vi "VI Graph.vi"() -> ()   [LabVIEW 2020, in "Grafik.lvlib"]
uses:
  Grafik.lvlib
  Visualisierungs Elemente/Zahlen-Ausgabefeld.ctl
  Visualisierungs Elemente/Auswahlfeld.ctl
  Visualisierungs Elemente/Button.ctl
  Aktionen Konfig Diagramme.ctl
  FT-IR/FGV FT-IR Gasliste Aktionen.ctl
  Gaszuordnung AO/FGV Gaszuordnung Gas-Auswahl Aktion.ctl
  Messdaten/Aktionen FGV Messdaten.ctl
  FT-IR/FGV FT-IR Parameter.vi
  FT-IR/FT-IR.lvlib
  Messdaten/Messdaten.lvlib
  Allgemein/allgemeine Sub-VIs.lvlib
  Gaszuordnung AO/Gaszuordnung AO.lvlib
panel:
  in  "Zoom deaktivieren":T1 caption="Graphen löschen"
  out "Mwert 6":sgl format="%.3f"
  out "PMwert 6":sgl format="%.3f"
  out "Mwert 5":sgl format="%.3f"
  out "PMwert 5":sgl format="%.3f"
  out "Mwert 4":sgl format="%.3f"
  out "PMwert 4":sgl format="%.3f"
  out "Mwert 3":sgl format="%.3f"
  out "PMwert 3":sgl format="%.3f"
  out "Mwert 2":sgl format="%.3f"
  out "PMwert 2":sgl format="%.3f"
  out "Mwert":sgl format="%.3f"
  out "PMwert":sgl format="%.3f"
  in  "Graphen löschen":T1
  in  "Konfig":T1
  out "Wert 6":T2 caption="Konzentration" format="%#.3f"
  out "Wert 5":T2 caption="Konzentration" format="%#.3f"
  in  "Gas 6":T3=1 items=["NO (3000) LP 191C", "NO2 (150) LP 191C (1of2)", "NO2 (2000) LP 191C (2of2)", "N2O (300) LP 191C (1of2)", "NH3 (300) LP 191C (1of2)", "NH3 (900,3000) LP 191C (2of2)", "HNCO (400) 191C", "H2O% (30) LP 191C", "Formaldehyde (70,500) LP 191C", "CO2 low% (4) LP 191C (2of2)", "CO2% (20) LP 191C (1of2)", "CO (700) LP 191C (1of3)", "CO% (1) LP 191C (2of3)", "Propylene (1000) LP 191C", "Aromatic HC C7 (500) LP 191C", "Ethylene (1000) LP 191C", "CH4 (250) LP 191C (1of2)", "CH4 (5000) LP 191C (2of2)", "Ethane (1000) LP 191C", "Acetylene (1000) LP 191C", "HNO2 (20) 191C", "MeOH (1000) 191C", "CO% (10) LP 191C (3of3)", "Formic Acid (100) 191C", "SO2 (500) LP 191C", "Acetaldehyde (1000) LP 191C", "COS (100) LP 191C", "1,3 butadiene (100) LP 191C", "Oil as Octane (200) LP 191C", "N2O (1000) LP 191C (2of2)", "Propane (200) LP 191C", "NO2 autorange (2000)", "CO autorange (100000)", "CH4 autorange (5000)", "NH3 autorange (3000)", "NOx autorange (3000)", "HCD (10000)", "NMHCD (10000)", "CO2% autorange (20)", "H2Oppm (300000)", "N2O autorange (1000)", "NMNEHCD (3000)", "Temp. Gascell", "Pressure Gascell", "sBeam@2500", "Temp. HL to FT-IR", "Temp. HL Extern SP1", "Outlet Temp FT-IR", "Temp. Cabinet", "Constant 0", "Constant 50", "Constant 100", "AK DUMMY"]
  in  "Gas 5":T3=1 items=["NO (3000) LP 191C", "NO2 (150) LP 191C (1of2)", "NO2 (2000) LP 191C (2of2)", "N2O (300) LP 191C (1of2)", "NH3 (300) LP 191C (1of2)", "NH3 (900,3000) LP 191C (2of2)", "HNCO (400) 191C", "H2O% (30) LP 191C", "Formaldehyde (70,500) LP 191C", "CO2 low% (4) LP 191C (2of2)", "CO2% (20) LP 191C (1of2)", "CO (700) LP 191C (1of3)", "CO% (1) LP 191C (2of3)", "Propylene (1000) LP 191C", "Aromatic HC C7 (500) LP 191C", "Ethylene (1000) LP 191C", "CH4 (250) LP 191C (1of2)", "CH4 (5000) LP 191C (2of2)", "Ethane (1000) LP 191C", "Acetylene (1000) LP 191C", "HNO2 (20) 191C", "MeOH (1000) 191C", "CO% (10) LP 191C (3of3)", "Formic Acid (100) 191C", "SO2 (500) LP 191C", "Acetaldehyde (1000) LP 191C", "COS (100) LP 191C", "1,3 butadiene (100) LP 191C", "Oil as Octane (200) LP 191C", "N2O (1000) LP 191C (2of2)", "Propane (200) LP 191C", "NO2 autorange (2000)", "CO autorange (100000)", "CH4 autorange (5000)", "NH3 autorange (3000)", "NOx autorange (3000)", "HCD (10000)", "NMHCD (10000)", "CO2% autorange (20)", "H2Oppm (300000)", "N2O autorange (1000)", "NMNEHCD (3000)", "Temp. Gascell", "Pressure Gascell", "sBeam@2500", "Temp. HL to FT-IR", "Temp. HL Extern SP1", "Outlet Temp FT-IR", "Temp. Cabinet", "Constant 0", "Constant 50", "Constant 100", "AK DUMMY"]
  in  "Gas 2":T3=1 items=["NO (3000) LP 191C", "NO2 (150) LP 191C (1of2)", "NO2 (2000) LP 191C (2of2)", "N2O (300) LP 191C (1of2)", "NH3 (300) LP 191C (1of2)", "NH3 (900,3000) LP 191C (2of2)", "HNCO (400) 191C", "H2O% (30) LP 191C", "Formaldehyde (70,500) LP 191C", "CO2 low% (4) LP 191C (2of2)", "CO2% (20) LP 191C (1of2)", "CO (700) LP 191C (1of3)", "CO% (1) LP 191C (2of3)", "Propylene (1000) LP 191C", "Aromatic HC C7 (500) LP 191C", "Ethylene (1000) LP 191C", "CH4 (250) LP 191C (1of2)", "CH4 (5000) LP 191C (2of2)", "Ethane (1000) LP 191C", "Acetylene (1000) LP 191C", "HNO2 (20) 191C", "MeOH (1000) 191C", "CO% (10) LP 191C (3of3)", "Formic Acid (100) 191C", "SO2 (500) LP 191C", "Acetaldehyde (1000) LP 191C", "COS (100) LP 191C", "1,3 butadiene (100) LP 191C", "Oil as Octane (200) LP 191C", "N2O (1000) LP 191C (2of2)", "Propane (200) LP 191C", "NO2 autorange (2000)", "CO autorange (100000)", "CH4 autorange (5000)", "NH3 autorange (3000)", "NOx autorange (3000)", "HCD (10000)", "NMHCD (10000)", "CO2% autorange (20)", "H2Oppm (300000)", "N2O autorange (1000)", "NMNEHCD (3000)", "Temp. Gascell", "Pressure Gascell", "sBeam@2500", "Temp. HL to FT-IR", "Temp. HL Extern SP1", "Outlet Temp FT-IR", "Temp. Cabinet", "Constant 0", "Constant 50", "Constant 100", "AK DUMMY"]
  out "Wert 2":T2 caption="Konzentration" format="%#.3f"
  in  "Gas 4":T3=1 items=["NO (3000) LP 191C", "NO2 (150) LP 191C (1of2)", "NO2 (2000) LP 191C (2of2)", "N2O (300) LP 191C (1of2)", "NH3 (300) LP 191C (1of2)", "NH3 (900,3000) LP 191C (2of2)", "HNCO (400) 191C", "H2O% (30) LP 191C", "Formaldehyde (70,500) LP 191C", "CO2 low% (4) LP 191C (2of2)", "CO2% (20) LP 191C (1of2)", "CO (700) LP 191C (1of3)", "CO% (1) LP 191C (2of3)", "Propylene (1000) LP 191C", "Aromatic HC C7 (500) LP 191C", "Ethylene (1000) LP 191C", "CH4 (250) LP 191C (1of2)", "CH4 (5000) LP 191C (2of2)", "Ethane (1000) LP 191C", "Acetylene (1000) LP 191C", "HNO2 (20) 191C", "MeOH (1000) 191C", "CO% (10) LP 191C (3of3)", "Formic Acid (100) 191C", "SO2 (500) LP 191C", "Acetaldehyde (1000) LP 191C", "COS (100) LP 191C", "1,3 butadiene (100) LP 191C", "Oil as Octane (200) LP 191C", "N2O (1000) LP 191C (2of2)", "Propane (200) LP 191C", "NO2 autorange (2000)", "CO autorange (100000)", "CH4 autorange (5000)", "NH3 autorange (3000)", "NOx autorange (3000)", "HCD (10000)", "NMHCD (10000)", "CO2% autorange (20)", "H2Oppm (300000)", "N2O autorange (1000)", "NMNEHCD (3000)", "Temp. Gascell", "Pressure Gascell", "sBeam@2500", "Temp. HL to FT-IR", "Temp. HL Extern SP1", "Outlet Temp FT-IR", "Temp. Cabinet", "Constant 0", "Constant 50", "Constant 100", "AK DUMMY"]
  in  "Gas 1":T3 items=["NO (3000) LP 191C", "NO2 (150) LP 191C (1of2)", "NO2 (2000) LP 191C (2of2)", "N2O (300) LP 191C (1of2)", "NH3 (300) LP 191C (1of2)", "NH3 (900,3000) LP 191C (2of2)", "HNCO (400) 191C", "H2O% (30) LP 191C", "Formaldehyde (70,500) LP 191C", "CO2 low% (4) LP 191C (2of2)", "CO2% (20) LP 191C (1of2)", "CO (700) LP 191C (1of3)", "CO% (1) LP 191C (2of3)", "Propylene (1000) LP 191C", "Aromatic HC C7 (500) LP 191C", "Ethylene (1000) LP 191C", "CH4 (250) LP 191C (1of2)", "CH4 (5000) LP 191C (2of2)", "Ethane (1000) LP 191C", "Acetylene (1000) LP 191C", "HNO2 (20) 191C", "MeOH (1000) 191C", "CO% (10) LP 191C (3of3)", "Formic Acid (100) 191C", "SO2 (500) LP 191C", "Acetaldehyde (1000) LP 191C", "COS (100) LP 191C", "1,3 butadiene (100) LP 191C", "Oil as Octane (200) LP 191C", "N2O (1000) LP 191C (2of2)", "Propane (200) LP 191C", "NO2 autorange (2000)", "CO autorange (100000)", "CH4 autorange (5000)", "NH3 autorange (3000)", "NOx autorange (3000)", "HCD (10000)", "NMHCD (10000)", "CO2% autorange (20)", "H2Oppm (300000)", "N2O autorange (1000)", "NMNEHCD (3000)", "Temp. Gascell", "Pressure Gascell", "sBeam@2500", "Temp. HL to FT-IR", "Temp. HL Extern SP1", "Outlet Temp FT-IR", "Temp. Cabinet", "Constant 0", "Constant 50", "Constant 100", "AK DUMMY"]
  out "Wert 1":T2 caption="Konzentration" format="%#.3f"
  out "Wert 4":T2 caption="Konzentration" format="%#.3f"
  out "Wert 3":T2 caption="Konzentration" format="%#.3f"
  in  "Gas 3":T3=1 items=["NO (3000) LP 191C", "NO2 (150) LP 191C (1of2)", "NO2 (2000) LP 191C (2of2)", "N2O (300) LP 191C (1of2)", "NH3 (300) LP 191C (1of2)", "NH3 (900,3000) LP 191C (2of2)", "HNCO (400) 191C", "H2O% (30) LP 191C", "Formaldehyde (70,500) LP 191C", "CO2 low% (4) LP 191C (2of2)", "CO2% (20) LP 191C (1of2)", "CO (700) LP 191C (1of3)", "CO% (1) LP 191C (2of3)", "Propylene (1000) LP 191C", "Aromatic HC C7 (500) LP 191C", "Ethylene (1000) LP 191C", "CH4 (250) LP 191C (1of2)", "CH4 (5000) LP 191C (2of2)", "Ethane (1000) LP 191C", "Acetylene (1000) LP 191C", "HNO2 (20) 191C", "MeOH (1000) 191C", "CO% (10) LP 191C (3of3)", "Formic Acid (100) 191C", "SO2 (500) LP 191C", "Acetaldehyde (1000) LP 191C", "COS (100) LP 191C", "1,3 butadiene (100) LP 191C", "Oil as Octane (200) LP 191C", "N2O (1000) LP 191C (2of2)", "Propane (200) LP 191C", "NO2 autorange (2000)", "CO autorange (100000)", "CH4 autorange (5000)", "NH3 autorange (3000)", "NOx autorange (3000)", "HCD (10000)", "NMHCD (10000)", "CO2% autorange (20)", "H2Oppm (300000)", "N2O autorange (1000)", "NMNEHCD (3000)", "Temp. Gascell", "Pressure Gascell", "sBeam@2500", "Temp. HL to FT-IR", "Temp. HL Extern SP1", "Outlet Temp FT-IR", "Temp. Cabinet", "Constant 0", "Constant 50", "Constant 100", "AK DUMMY"]
  out "Graph1":waveform(dbl)[](graph)
  out "Graph 3":waveform(dbl)[](graph)
  out "Graph 2":waveform(dbl)[](graph)
  out "Graph 4":waveform(dbl)[](graph)
  out "Graph 6":waveform(dbl)[](graph)
  out "Graph 5":waveform(dbl)[](graph)
  # "Grafik"
  # "Grafik 4"
  # "Grafik 1"
  # "Grafik 2"
  # "Grafik 5"
  # "Grafik 6"
  # "Grafik 3"
  # "±"
  # "x"
  # "±"
  # "x"
  # "±"
  # "x"
  # "±"
  # "x"
  # "±"
  # "x"
  # "±"
  # "x"
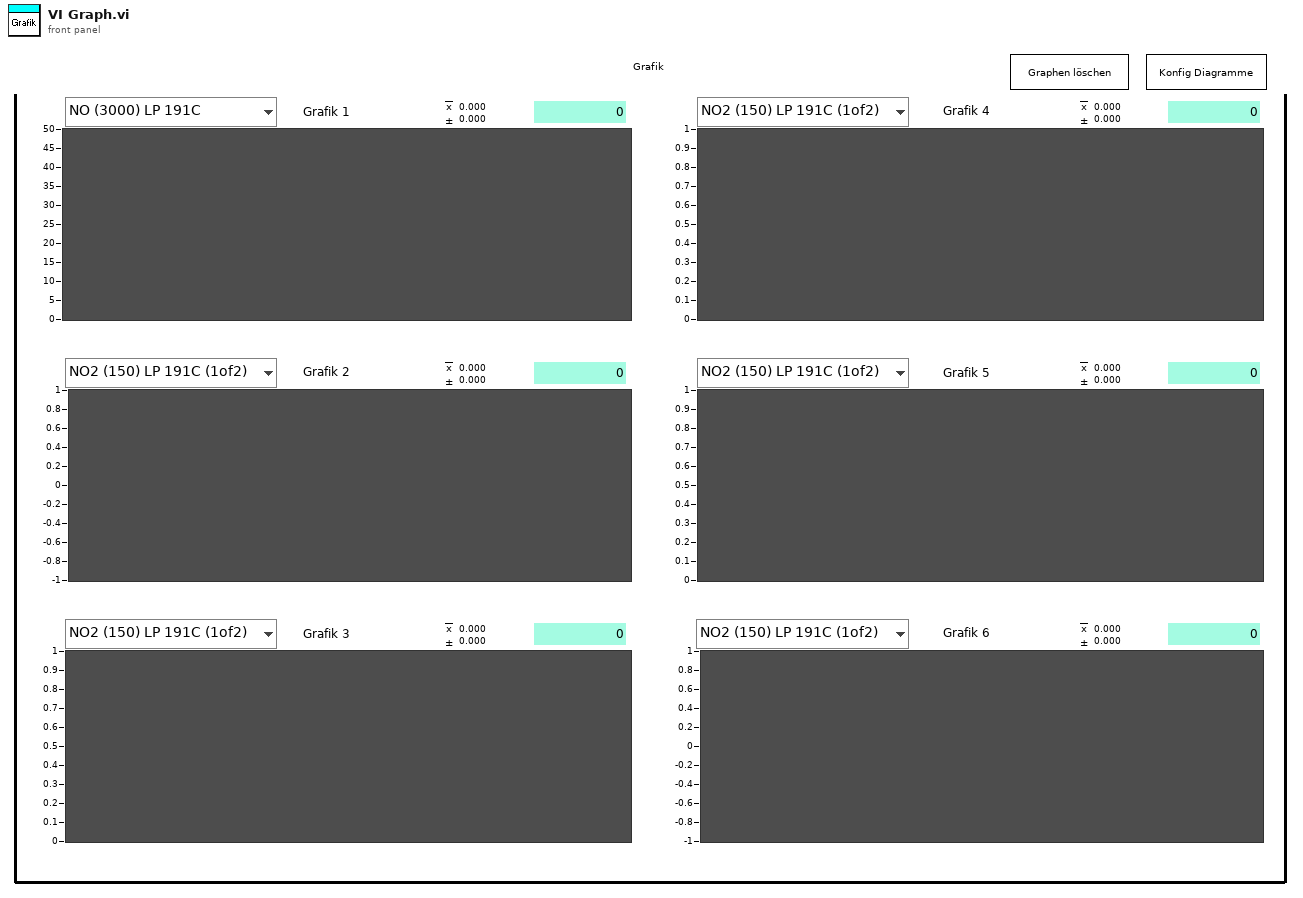
[diagram p1: front panel]
types:
  T1 = typedef "Button.ctl" = bool
  T2 = typedef "Zahlen-Ausgabefeld.ctl" = sgl
  T3 = typedef "Auswahlfeld.ctl" = u16
  T4 = typedef "Gaszuordnung AO.lvlib/FGV Gaszuordnung Gas-Auswahl Aktion.ctl" = enum16{"Lesen", "AO Auswahl", "Graph Auswahl", "aktiver Graph", "laden", "speichern"}
  T5 = typedef "FT-IR.lvlib/FGV FT-IR Gasliste Aktionen.ctl" = enum16{"lesen", "Gasliste FT-IR", "Gasliste ausgelesen", "laden", "speichern", "löschen"}
  T6 = typedef "Grafik.lvlib/Aktionen Konfig Diagramme.ctl" = enum16{"lesen", "laden", "speichern", "X Auto Scale", "Y Auto Scale", "Anzeigedauer", "Y MIN", "Y MAX", "Referenzen", "Werteanzahl", "Autoscale einzeln"}
  T7 = typedef "Zahlen-Eingabefeld.ctl" = sgl
  T8 = cluster{"Y Anzeige MIN 1":T7, "Y Anzeige MIN 2":T7, "Y Anzeige MIN 3":T7, "Y Anzeige MIN 4":T7, "Y Anzeige MIN 5":T7, "Y Anzeige MIN 6":T7}
  T9 = cluster{"Y Anzeige MAX 1":T7, "Y Anzeige MAX 2":T7, "Y Anzeige MAX 3":T7, "Y Anzeige MAX 4":T7, "Y Anzeige MAX 5":T7, "Y Anzeige MAX 6":T7}
  T10 = typedef "String - Ausgabefeld.ctl" = string
  T11 = typedef "Grafik.lvlib/Graphen Auswahl.ctl" = u16[]
  T12 = cluster{"Graphen[0]":u16, "Graphen[1]":u16, "Graphen[2]":u16, "Graphen[3]":u16, "Graphen[4]":u16, "Graphen[5]":u16}
  T13 = typedef "Messdaten.lvlib/Aktionen FGV Messdaten.ctl" = enum16{"lesen", "schreiben", "löschen", "Mittelwerte", "Komponente"}
  T14 = cluster{"[0]":waveform(dbl), "[1]":waveform(dbl), "[2]":waveform(dbl)}
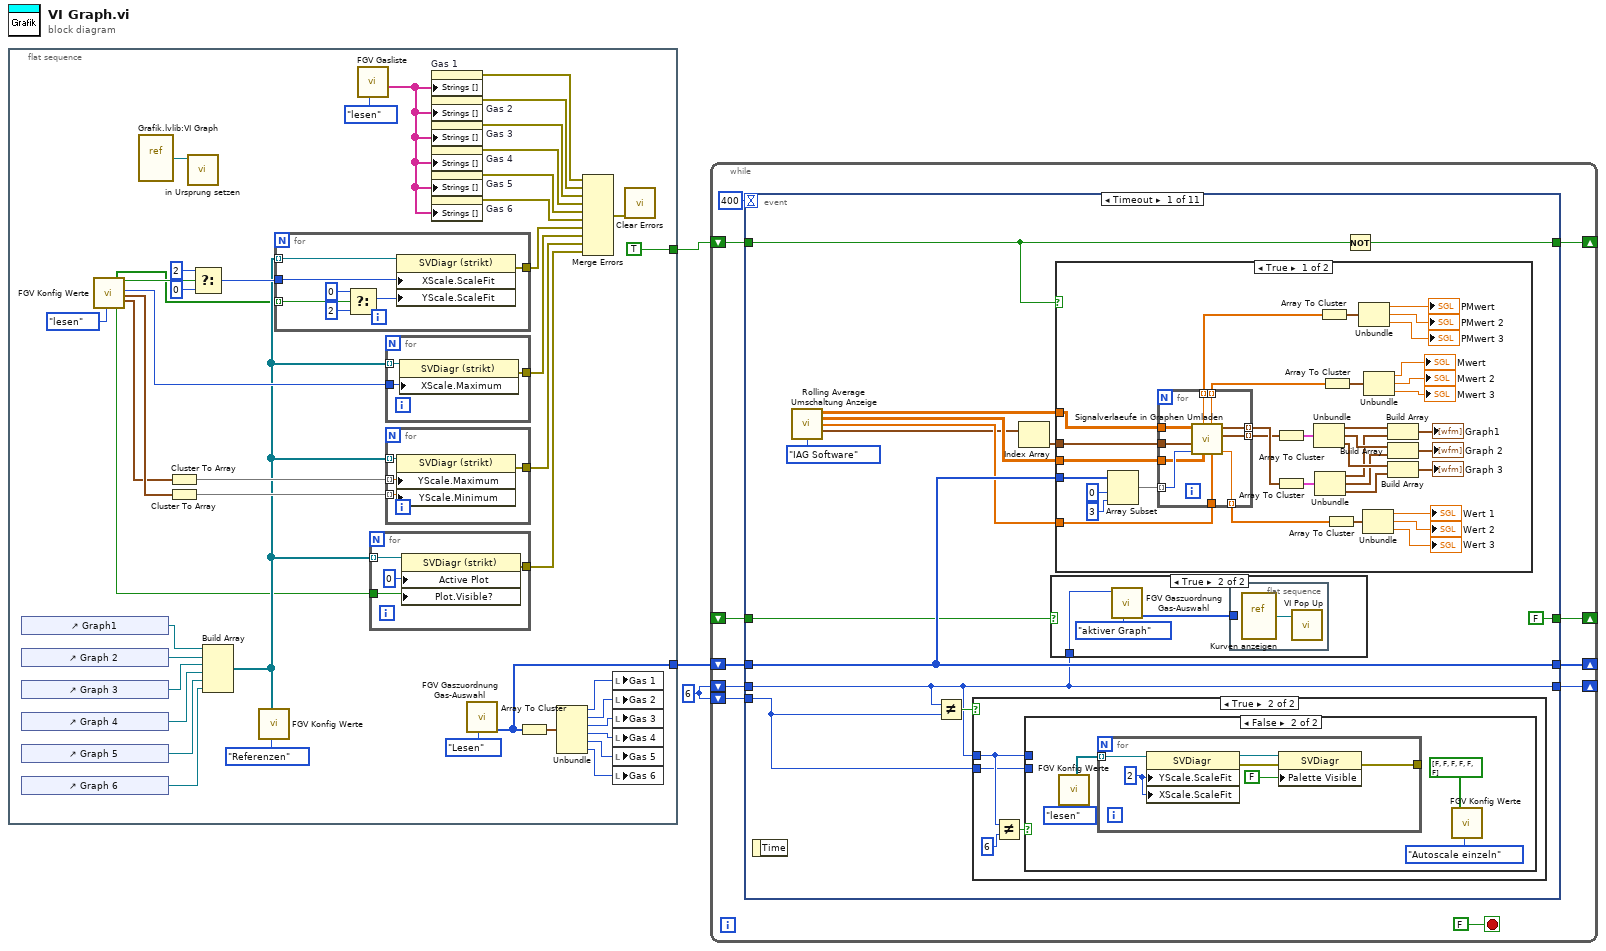
[diagram p0: block diagram]
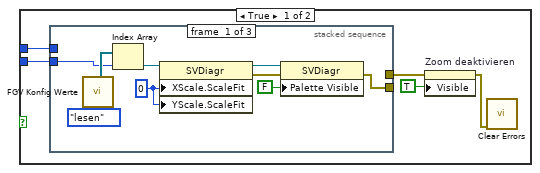
[diagram p4: hidden frame]
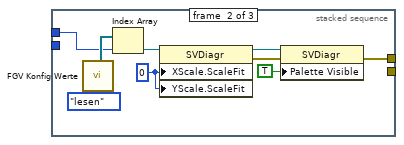
[diagram p5: hidden frame]
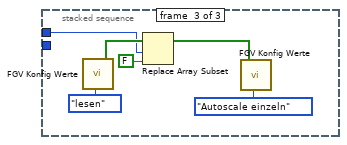
[diagram p6: hidden frame]
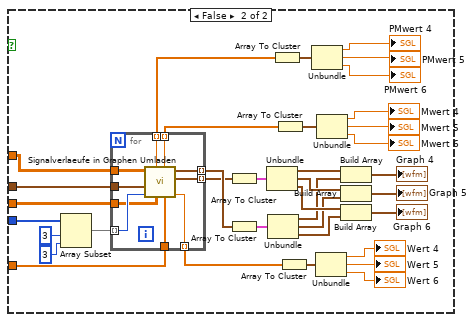
[diagram p7: hidden frame]
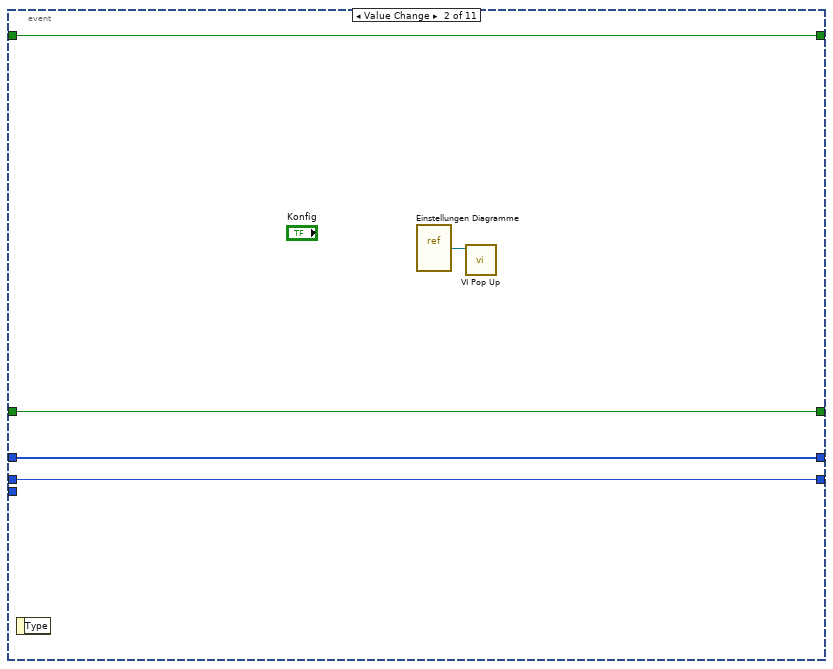
[diagram p8: hidden frame]
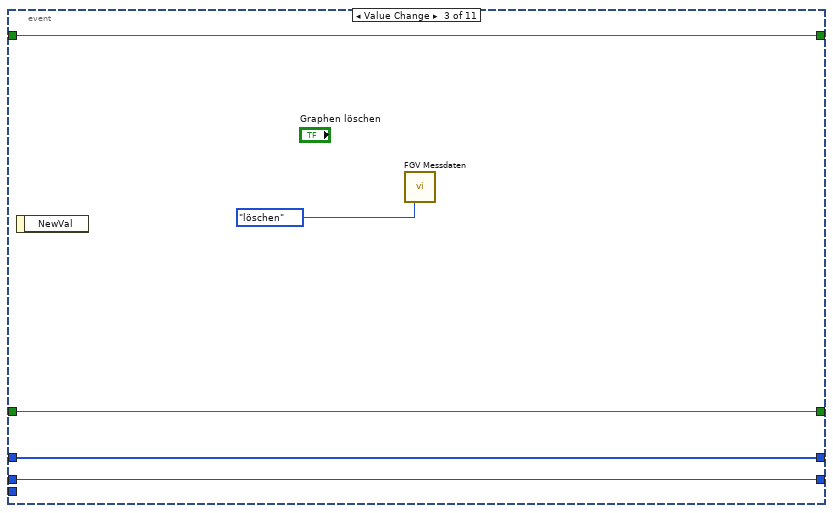
[diagram p9: hidden frame]
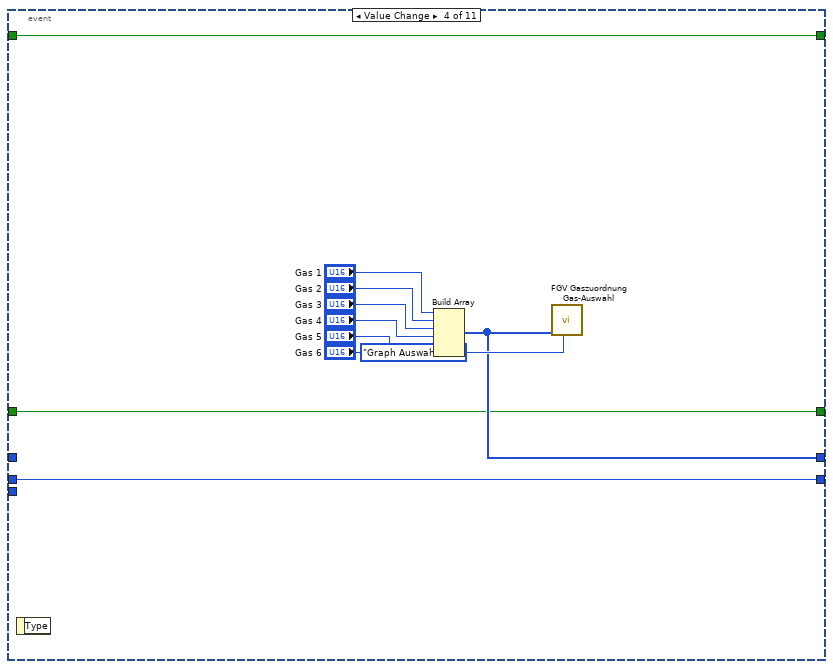
[diagram p10: hidden frame]
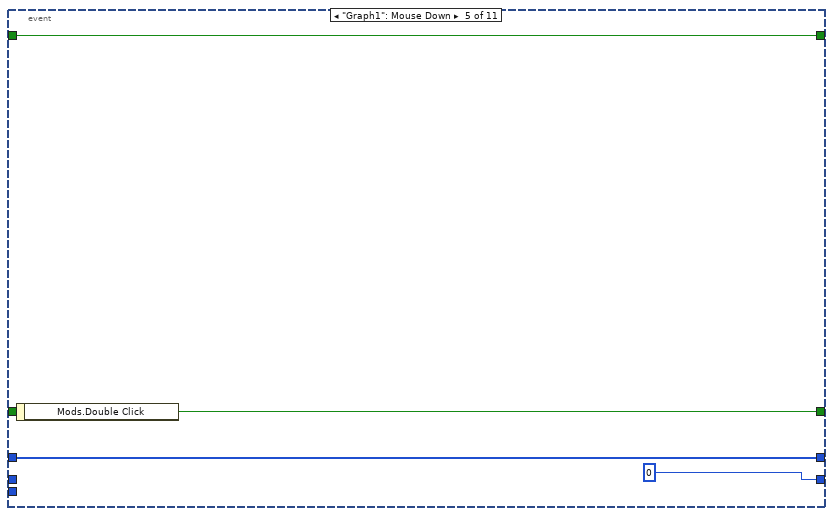
[diagram p11: hidden frame]
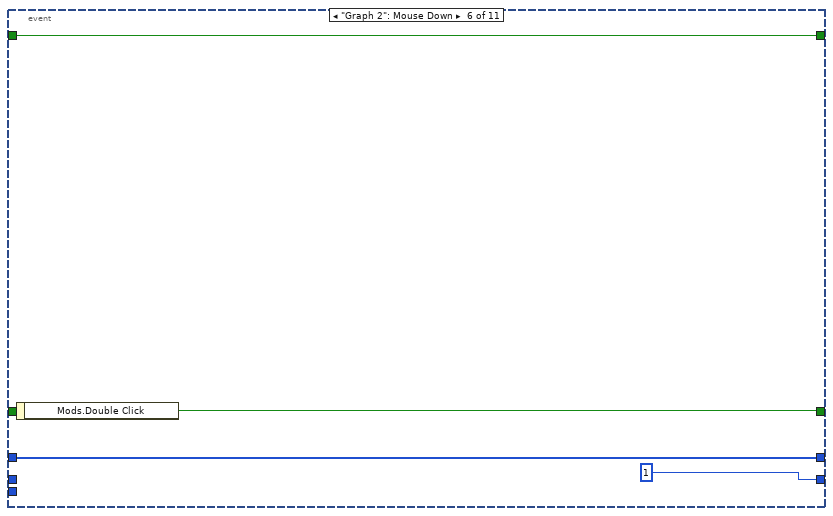
[diagram p12: hidden frame]
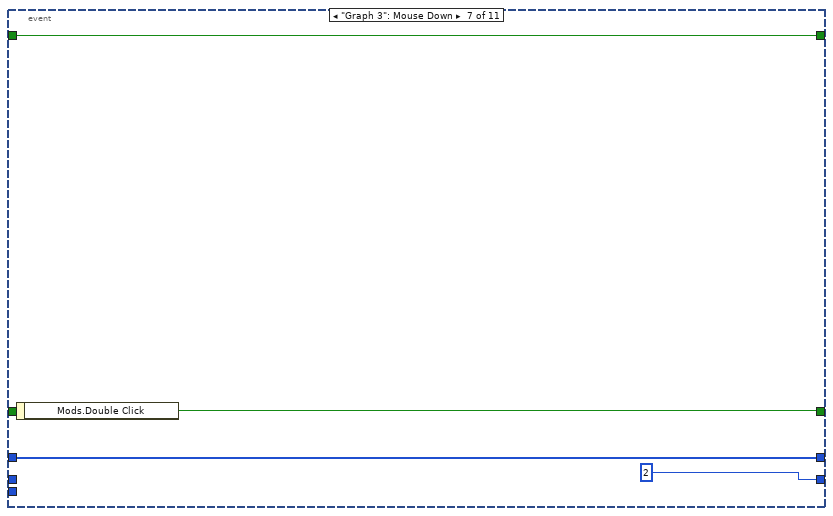
[diagram p13: hidden frame]
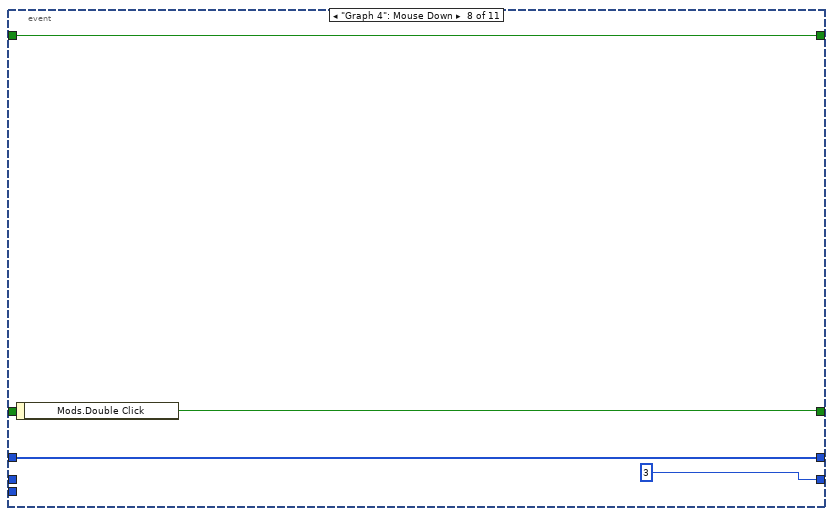
[diagram p14: hidden frame]
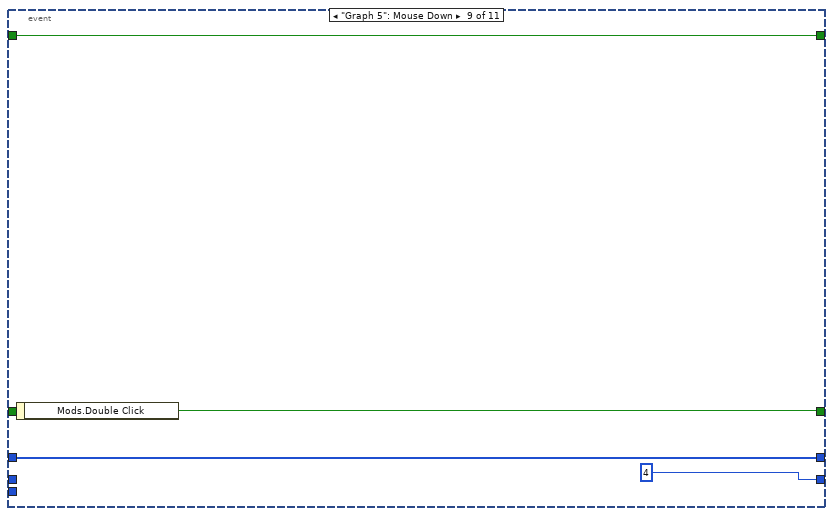
[diagram p15: hidden frame]
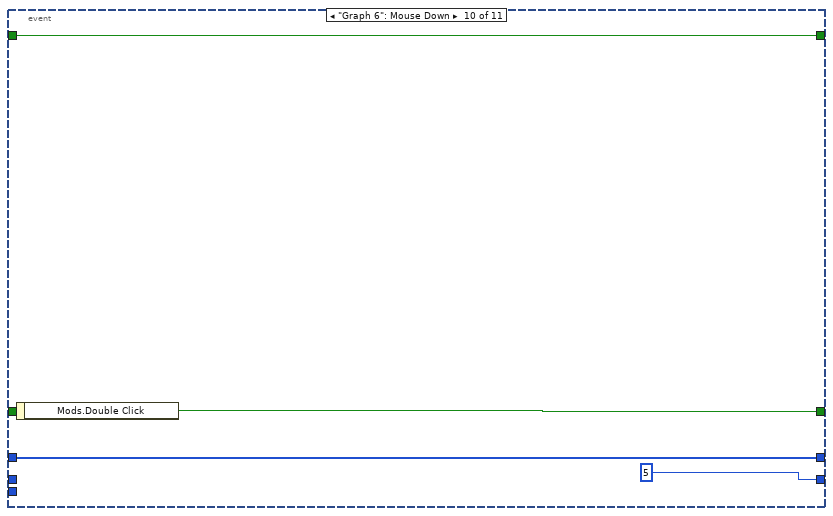
[diagram p16: hidden frame]
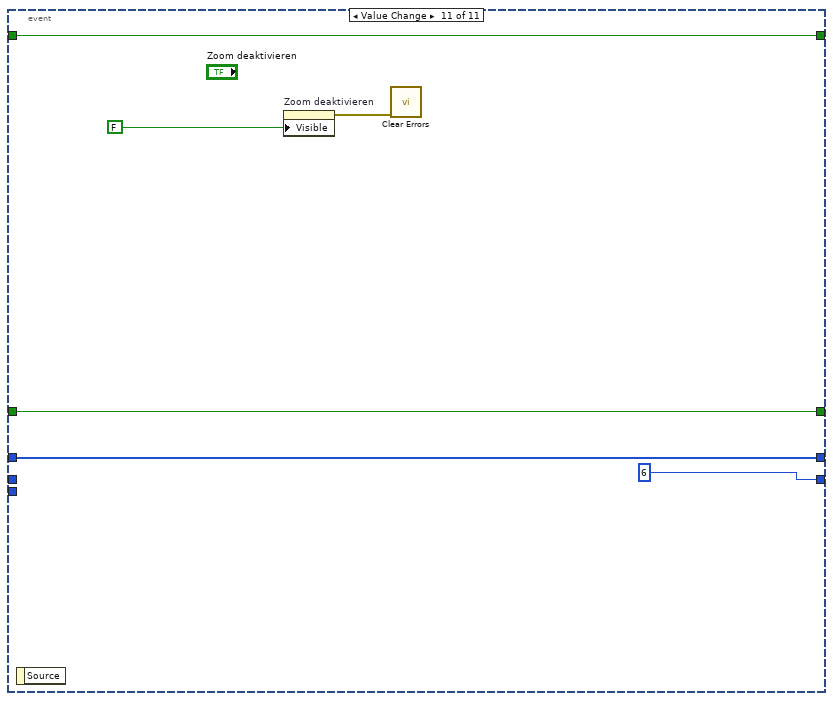
[diagram p17: hidden frame]
diagram:
  w1 = 6 ("t")
  n1 = flat-sequence {
    tunnel: [w6] -> w3
    tunnel: [TRUE] -> w2
    frame #0 {
      n2 = control-ref of="Graph1"() -> (w29:refnum<vi>)
      n3 = control-ref of="Graph 2"() -> (w28:refnum<vi>)
      n4 = control-ref of="Graph 3"() -> (w27:refnum<vi>)
      n5 = control-ref of="Graph 4"() -> (w26:refnum<vi>)
      n6 = control-ref of="Graph 5"() -> (w25:refnum<vi>)
      n7 = control-ref of="Graph 6"() -> (w24:refnum<vi>)
      n8 = call "FGV Konfig Werte.vi"("Aktionen"=Aktionen_Konfig_Diagramme."lesen" ("Aktionen Konfig Diagramme")) -> ("Autoscale einzeln"=w4:bool[], "Mittelwertanzeige"=w22:bool, "Auto Scale X"=w36:bool, "X Anzeigedauer"=w35:T3, "Y Anzeige MIN"=w34:T8, "Y Anzeige MAX"=w33:T9)  [unwired: 10 in, 3 out]
      n9 = vi-ref "Grafik.lvlib:VI Graph.vi"() -> (w5:refnum<vi>)
      n10 = Cluster To Array(cluster=w33) -> (array=w32:T7[])
      n11 = Cluster To Array(cluster=w34) -> (array=w31:T7[])
      n12 = call "in Ursprung setzen.vi"("VI Referenz"=w5) -> ()  [unwired: 10 in, 1 out]
      n13 = Select(t=u8 2 ("X-Achse.Achsenanpassung"), s=w36, f=u8 0 ("X-Achse.Achsenanpassung")) -> (s? t:f=w39:u8)
      n14 = Build Array(w29, w28, w27, w26, w25, w24) -> (w23:refnum<vi>[])
      n15 = call "FGV Konfig Werte.vi"("Referenzen"=w23, "Aktionen"=Aktionen_Konfig_Diagramme."Referenzen" ("Aktionen Konfig Diagramme")) -> ()  [unwired: 9 in, 9 out]
      n16 = for {
        tunnel: w39 -> [w65]
        tunnel: w23 -> [w64] mode=indexing
        tunnel: [w63] -> w13
        tunnel: w4 -> [w59] mode=indexing
        n17 = Select(t=u8 0 ("X-Achse.Achsenanpassung"), s=w59, f=u8 2 ("X-Achse.Achsenanpassung")) -> (s? t:f=w60:u8)
        n18 = property on="Eigenschaftsknoten" class="SVDiagr (strikt)"(reference=w64, "XScale.ScaleFit"=w65, "YScale.ScaleFit"=w60) -> (error out=w63:errorcluster)  [unwired: 1 in, 1 out]
      }
      n19 = call "FGV Gasliste.vi"("Aktionen"=FGV_FT-IR_Gasliste_Aktionen."lesen") -> ("Aktuelle Gasliste gesamt"=w20:T10[])  [unwired: 8 in, 2 out]
      n20 = for {
        tunnel: w23 -> [w51] mode=indexing
        tunnel: w22 -> [w49]
        tunnel: [w48] -> w10
        n21 = property class="SVDiagr (strikt)"(reference=w51, "Active Plot"=u32 0 ("Aktiver Plot"), "Plot.Visible?"=w49) -> (error out=w48:errorcluster)  [unwired: 1 in, 1 out]
      }
      n22 = for {
        tunnel: w35 -> [w54]
        tunnel: w23 -> [w53] mode=indexing
        tunnel: [w52] -> w12
        n23 = property on="Eigenschaftsknoten" class="SVDiagr (strikt)"(reference=w53, "XScale.Maximum"=w54) -> (error out=w52:errorcluster)  [unwired: 1 in, 1 out]
      }
      n24 = for {
        tunnel: w32 -> [w58] mode=indexing
        tunnel: w31 -> [w57] mode=indexing
        tunnel: w23 -> [w56] mode=indexing
        tunnel: [w55] -> w11
        n25 = property on="Eigenschaftsknoten" class="SVDiagr (strikt)"(reference=w56, "YScale.Maximum"=w58, "YScale.Minimum"=w57) -> (error out=w55:errorcluster)  [unwired: 1 in, 1 out]
      }
      n26 = property on="Gas 1" class="Ring (strikt)"("Strings []"=w20) -> (error out=w19:errorcluster)  [unwired: 2 in, 1 out]
      n27 = property on="Gas 2" class="Ring (strikt)"("Strings []"=w20) -> (error out=w18:errorcluster)  [unwired: 2 in, 1 out]
      n28 = property on="Gas 3" class="Ring (strikt)"("Strings []"=w20) -> (error out=w17:errorcluster)  [unwired: 2 in, 1 out]
      n29 = property on="Gas 4" class="Ring (strikt)"("Strings []"=w20) -> (error out=w16:errorcluster)  [unwired: 2 in, 1 out]
      n30 = property on="Gas 5" class="Ring (strikt)"("Strings []"=w20) -> (error out=w15:errorcluster)  [unwired: 2 in, 1 out]
      n31 = property on="Gas 6" class="Ring (strikt)"("Strings []"=w20) -> (error out=w14:errorcluster)  [unwired: 2 in, 1 out]
      n32 = call "FGV Gaszuordnung Gas-Auswahl.vi"("Aktion"=FGV_Gaszuordnung_Gas-Auswahl_Aktion."Lesen") -> ("Graphen"=w6:T11)  [unwired: 8 in, 2 out]
      n33 = Array To Cluster(array=w6) -> (cluster=w47:T12)
      n34 = Unbundle(w47) -> ("Graphen[0]"=w30:u16, "Graphen[1]"=w46:u16, "Graphen[2]"=w45:u16, "Graphen[3]"=w44:u16, "Graphen[4]"=w43:u16, "Graphen[5]"=w42:u16)
      n35 = Merge Errors(w19, w18, w17, w16, w15, w14, w13, w12, w11, w10) -> (w9:errorcluster)
      n36 = local write "Gas 1"(w30) -> ()
      n37 = local write "Gas 2"(w46) -> ()
      n38 = local write "Gas 3"(w45) -> ()
      n39 = local write "Gas 4"(w44) -> ()
      n40 = local write "Gas 5"(w43) -> ()
      n41 = local write "Gas 6"(w42) -> ()
      n42 = call <vilib>:"Clear Errors.vi"("error in (no error)"=w9) -> ()  [unwired: 5 in, 2 out]
    }
  }
  n43 = while {
    shift-right: [w75] -> _
    shift-left: w3 -> [w74]
    shift-right: [w72] -> _
    shift-left: w2 -> [w71]
    shift-right: [w70] -> _
    shift-left: w1 -> [w69]
    shift-left: w1 -> [w68]
    shift-right: [w67] -> _
    shift-left: _ -> [w66]
    stop <- FALSE stop-if-true
    n44 = event shown="[0] Timeout" {
      selector: _ -> [_ _ _ _ _ _ _ _ _ _ _]
      dyn-events: _ -> [_ _ _ _ _ _ _ _ _ _ _]
      timeout: 400 -> [_ _ _ _ _ _ _ _ _ _ _]
      tunnel: w74 -> [w89 w234 w239 _ w253 w256 w261 w265 w268 w273 w278]
      tunnel: [w89 w234 w239 w243 w253 w256 w261 w265 w268 w273 w278] -> w75
      tunnel: w71 -> [w87 w232 w237 w242 w252 w257 w260 w264 w269 w272 w279]
      tunnel: [w88 w232 w237 w242 w252 w257 w260 w264 w269 w272 w279] -> w72
      tunnel: [w82 w231 w236 w241 0 1 2 3 4 5 6 ("t")] -> w70
      tunnel: w69 -> [w82 w231 w236 w241 _ _ _ _ _ _ _]
      tunnel: w68 -> [w85 _ _ _ _ _ _ _ _ _ _]
      tunnel: [FALSE ("Double Click") w230 w235 w240 w251 w255 w259 w263 w267 w271 w275] -> w67
      tunnel: w66 -> [w84 w230 w235 w240 _ _ _ _ _ _ w275]
      event Timeout {
        n45 = event-data() -> ()  [unwired: 1 in, 1 out]
        n46 = call "Rolling Average Umschaltung Anzeige.vi"("Aktion"=enum16{"AK", "IAG Software"}."IAG Software") -> ("Messdaten"=w81:sgl[][], "Mittelwertdaten"=w80:sgl[][], "Deviation"=w79:sgl[], "Zeitstempeln"=w78:timestamp[])  [unwired: 9 in, 2 out]
        n47 = Not Equal?(x=w82, y=w85) -> (x != y?=w86:bool)
        n48 = case shown="True" w86 {
          tunnel: w82 -> [_ w98]
          tunnel: w85 -> [_ w95]
          frame False {
          }
          frame True {
            n49 = Not Equal?(x=w98, y=6) -> (x != y?=w96:bool)
            n50 = case shown="False" w96 {
              tunnel: w98 -> [w102 _]
              tunnel: w95 -> [w103 _]
              frame True {
                n51 = stacked-sequence {
                  tunnel: w103 -> [w105 _ _]
                  tunnel: w102 -> [_ w114 w124]
                  tunnel: [_ w113 _] -> w99
                  tunnel: [w104 _ _] -> _
                  frame #0 {
                    w109 = u8 0 ("X-Achse.Achsenanpassung")
                    n52 = call "FGV Konfig Werte.vi"("Aktionen"=Aktionen_Konfig_Diagramme."lesen") -> ("Referenzen"=w111:refnum<vi>[])  [unwired: 10 in, 8 out]
                    n53 = Index Array(array=w111, index=w105) -> (element=w110:refnum<vi>)
                    n54 = property class="SVDiagr"(reference=w110, "XScale.ScaleFit"=w109, "YScale.ScaleFit"=w109) -> (reference out=w108:refnum<vi>, error out=w107:errorcluster)  [unwired: 1 in]
                    n55 = property class="SVDiagr"(reference=w108, error in=w107, "Palette Visible"=FALSE ("Palette:Sichtbar")) -> (error out=w104:errorcluster)  [unwired: 1 out]
                  }
                  frame #1 {
                    w118 = u8 0 ("X-Achse.Achsenanpassung")
                    n56 = call "FGV Konfig Werte.vi"("Aktionen"=Aktionen_Konfig_Diagramme."lesen") -> ("Referenzen"=w120:refnum<vi>[])  [unwired: 10 in, 8 out]
                    n57 = Index Array(array=w120, index=w114) -> (element=w119:refnum<vi>)
                    n58 = property class="SVDiagr"(reference=w119, "XScale.ScaleFit"=w118, "YScale.ScaleFit"=w118) -> (reference out=w117:refnum<vi>, error out=w116:errorcluster)  [unwired: 1 in]
                    n59 = property class="SVDiagr"(reference=w117, error in=w116, "Palette Visible"=TRUE ("Palette:Sichtbar")) -> (error out=w113:errorcluster)  [unwired: 1 out]
                  }
                  frame #2 {
                    n60 = call "FGV Konfig Werte.vi"("Aktionen"=Aktionen_Konfig_Diagramme."lesen") -> ("Autoscale einzeln"=w126:bool[])  [unwired: 10 in, 8 out]
                    n61 = Replace Array Subset(array=w126, new element=FALSE ("Neues Element/Teil-Array"), index=w124) -> (w122:bool[])
                    n62 = call "FGV Konfig Werte.vi"("Autoscale einzeln"=w122, "Aktionen"=Aktionen_Konfig_Diagramme."Autoscale einzeln") -> ()  [unwired: 9 in, 9 out]
                  }
                }
                n63 = property on="Zoom deaktivieren" class="Bool."(error in=w99, "Visible"=TRUE) -> (error out=w100:errorcluster)  [unwired: 1 in, 1 out]
                n64 = call <vilib>:"Clear Errors.vi"("error in (no error)"=w100) -> ()  [unwired: 5 in, 2 out]
              }
              frame False {
                n65 = call "FGV Konfig Werte.vi"("Aktionen"=Aktionen_Konfig_Diagramme."lesen") -> ("Referenzen"=w130:refnum<vi>[])  [unwired: 10 in, 8 out]
                n66 = for {
                  tunnel: [w136] -> _
                  tunnel: w130 -> [w135] mode=indexing
                  w134 = u8 2 ("Y-Achse.Achsenanpassung")
                  n67 = property class="SVDiagr"(reference=w135, "YScale.ScaleFit"=w134, "XScale.ScaleFit"=w134) -> (reference out=w133:refnum<vi>, error out=w132:errorcluster)  [unwired: 1 in]
                  n68 = property class="SVDiagr"(reference=w133, error in=w132, "Palette Visible"=FALSE ("Palette:Sichtbar")) -> (error out=w136:errorcluster)  [unwired: 1 out]
                }
                n69 = call "FGV Konfig Werte.vi"("Autoscale einzeln"=bool[] [FALSE, FALSE, FALSE, FALSE, FALSE, FALSE], "Aktionen"=Aktionen_Konfig_Diagramme."Autoscale einzeln") -> ()  [unwired: 9 in, 9 out]
              }
            }
          }
        }
        n70 = Index Array(array=w78) -> (element=w90:timestamp)  [unwired: 1 in]
        n71 = case shown="True" w84 {
          tunnel: w82 -> [_ w92]
          frame False {
          }
          frame True {
            n72 = call "FGV Gaszuordnung Gas-Auswahl.vi"("Aktion"=FGV_Gaszuordnung_Gas-Auswahl_Aktion."aktiver Graph", "aktiver Graph"=w92) -> ("Graphen"=w91:T11)  [unwired: 7 in, 2 out]
            n73 = flat-sequence {
              tunnel: w91 -> [_]
              frame #0 {
                n74 = vi-ref "Kurven anzeigen.vi"() -> (w94:refnum<vi>)
                n75 = call "VI Pop Up.vi"("VI Referenz"=w94) -> ()  [unwired: 10 in, 1 out]
              }
            }
          }
        }
        n76 = case shown="True" w87 {
          tunnel: w90 -> [w173 w219]
          tunnel: w79 -> [w172 w218]
          tunnel: w89 -> [w141 w198]
          tunnel: w81 -> [w144 w201]
          tunnel: w80 -> [w143 w200]
          frame True {
            n77 = Array Subset(array=w141, index=0 ("Index"), length=3 ("Länge")) -> (w142:T3[])
            n78 = for {
              tunnel: w142 -> [w183] mode=indexing
              tunnel: w144 -> [w182]
              tunnel: w173 -> [w181]
              tunnel: w143 -> [w174]
              tunnel: w172 -> [w180]
              tunnel: [w179] -> w138 mode=indexing
              tunnel: [w178] -> w166 mode=indexing
              tunnel: [w177] -> w167 mode=indexing
              tunnel: [w176] -> w152 mode=indexing
              tunnel: [w175] -> w148 mode=indexing
              n79 = call "Signalverlaeufe in Graphen Umladen.vi"("Deviation"=w180, "Mittelwertdaten"=w174, "Gas-Auswahl"=w183, "t0"=w181, "Werte"=w182) -> ("Konzentration"=w179:sgl, "Mittelwert"=w178:waveform(dbl), "Waveform"=w177:waveform(dbl), "aktuelle Mittelwert"=w176:sgl, "Deviation"=w175:sgl)  [unwired: 2 in]
            }
            n80 = Array To Cluster(array=w166) -> (cluster=w164:T14)
            n81 = Array To Cluster(array=w167) -> (cluster=w165:T14)
            n82 = Unbundle(w164) -> ("[0]"=w163:waveform(dbl), "[1]"=w162:waveform(dbl), "[2]"=w161:waveform(dbl))
            n83 = Unbundle(w165) -> ("[0]"=w157:waveform(dbl), "[1]"=w156:waveform(dbl), "[2]"=w155:waveform(dbl))
            n84 = Array To Cluster(array=w148) -> (cluster=w154:cluster{"[0]":sgl, "[1]":sgl, "[2]":sgl})
            n85 = Array To Cluster(array=w152) -> (cluster=w153:cluster{"[0]":sgl, "[1]":sgl, "[2]":sgl})
            n86 = Array To Cluster(array=w138) -> (cluster=w171:cluster{"[0]":sgl, "[1]":sgl, "[2]":sgl})
            n87 = Unbundle(w154) -> ("[0]"=→"PMwert":sgl, "[1]"=→"PMwert 2":sgl, "[2]"=→"PMwert 3":sgl)
            n88 = Unbundle(w171) -> ("[0]"=→"Wert 1":sgl, "[1]"=→"Wert 2":sgl, "[2]"=→"Wert 3":sgl)
            n89 = Unbundle(w153) -> ("[0]"=→"Mwert":sgl, "[1]"=→"Mwert 2":sgl, "[2]"=→"Mwert 3":sgl)
            n90 = Build Array(w163, w157) -> (→"Graph1":waveform(dbl)[])
            n91 = Build Array(w162, w156) -> (→"Graph 2":waveform(dbl)[])
            n92 = Build Array(w161, w155) -> (→"Graph 3":waveform(dbl)[])
          }
          frame False {
            n93 = Array Subset(array=w198, index=3 ("Index"), length=3 ("Länge")) -> (w199:T3[])
            n94 = for {
              tunnel: w199 -> [w229] mode=indexing
              tunnel: w201 -> [w228]
              tunnel: w219 -> [w227]
              tunnel: w200 -> [w226]
              tunnel: w218 -> [w225]
              tunnel: [w224] -> w217 mode=indexing
              tunnel: [w223] -> w214 mode=indexing
              tunnel: [w222] -> w215 mode=indexing
              tunnel: [w221] -> w203 mode=indexing
              tunnel: [w220] -> w202 mode=indexing
              n95 = call "Signalverlaeufe in Graphen Umladen.vi"("Deviation"=w225, "Mittelwertdaten"=w226, "Gas-Auswahl"=w229, "t0"=w227, "Werte"=w228) -> ("Konzentration"=w224:sgl, "Mittelwert"=w223:waveform(dbl), "Waveform"=w222:waveform(dbl), "aktuelle Mittelwert"=w221:sgl, "Deviation"=w220:sgl)  [unwired: 2 in]
            }
            n96 = Array To Cluster(array=w214) -> (cluster=w212:T14)
            n97 = Array To Cluster(array=w215) -> (cluster=w213:T14)
            n98 = Unbundle(w212) -> ("[0]"=w211:waveform(dbl), "[1]"=w210:waveform(dbl), "[2]"=w209:waveform(dbl))
            n99 = Unbundle(w213) -> ("[0]"=w208:waveform(dbl), "[1]"=w207:waveform(dbl), "[2]"=w206:waveform(dbl))
            n100 = Array To Cluster(array=w202) -> (cluster=w205:cluster{"[0]":sgl, "[1]":sgl, "[2]":sgl})
            n101 = Array To Cluster(array=w203) -> (cluster=w204:cluster{"[0]":sgl, "[1]":sgl, "[2]":sgl})
            n102 = Array To Cluster(array=w217) -> (cluster=w216:cluster{"[0]":sgl, "[1]":sgl, "[2]":sgl})
            n103 = Unbundle(w205) -> ("[0]"=→"PMwert 4":sgl, "[1]"=→"PMwert 5":sgl, "[2]"=→"PMwert 6":sgl)
            n104 = Unbundle(w216) -> ("[0]"=→"Wert 4":sgl, "[1]"=→"Wert 5":sgl, "[2]"=→"Wert 6":sgl)
            n105 = Unbundle(w204) -> ("[0]"=→"Mwert 4":sgl, "[1]"=→"Mwert 5":sgl, "[2]"=→"Mwert 6":sgl)
            n106 = Build Array(w211, w208) -> (→"Graph 4":waveform(dbl)[])
            n107 = Build Array(w210, w207) -> (→"Graph 5":waveform(dbl)[])
            n108 = Build Array(w209, w206) -> (→"Graph 6":waveform(dbl)[])
          }
        }
        n109 = Not(x=w87) -> (.not. x?=w88:bool)
      }
      event Value Change {
        n110 = event-data() -> ()  [unwired: 1 in, 1 out]
        n111 = vi-ref "Einstellungen Diagramme.vi"() -> (w233:refnum<vi>)
        n112 = call "VI Pop Up.vi"("VI Referenz"=w233) -> ()  [unwired: 10 in, 1 out]
      }
      event Value Change {
        n113 = event-data() -> ()  [unwired: 1 in, 1 out]
        n114 = call "FGV Messdaten.vi"("Aktionen"=Aktionen_FGV_Messdaten."löschen") -> ()  [unwired: 6 in, 9 out]
      }
      event Value Change {
        n115 = event-data() -> ()  [unwired: 1 in, 1 out]
        n116 = Build Array("Gas 1", "Gas 2", "Gas 3", "Gas 4", "Gas 5", "Gas 6") -> (w243:T3[])
        n117 = call "FGV Gaszuordnung Gas-Auswahl.vi"("Aktion"=FGV_Gaszuordnung_Gas-Auswahl_Aktion."Graph Auswahl", "Graphen"=w243) -> ()  [unwired: 7 in, 3 out]
      }
      event "Graph1": Mouse Down {
        n118 = event-data() -> ("Mods.Double Click"=w251:bool)  [unwired: 1 in]
      }
      event "Graph 2": Mouse Down {
        n119 = event-data() -> ("Mods.Double Click"=w255:bool)  [unwired: 1 in]
      }
      event "Graph 3": Mouse Down {
        n120 = event-data() -> ("Mods.Double Click"=w259:bool)  [unwired: 1 in]
      }
      event "Graph 4": Mouse Down {
        n121 = event-data() -> ("Mods.Double Click"=w263:bool)  [unwired: 1 in]
      }
      event "Graph 5": Mouse Down {
        n122 = event-data() -> ("Mods.Double Click"=w267:bool)  [unwired: 1 in]
      }
      event "Graph 6": Mouse Down {
        n123 = event-data() -> ("Mods.Double Click"=w271:bool)  [unwired: 1 in]
      }
      event Value Change {
        n124 = event-data() -> ()  [unwired: 1 in, 1 out]
        n125 = property on="Zoom deaktivieren" class="Bool."("Visible"=FALSE ("Sichtbar")) -> (error out=w276:errorcluster)  [unwired: 2 in, 1 out]
        n126 = call <vilib>:"Clear Errors.vi"("error in (no error)"=w276) -> ()  [unwired: 5 in, 2 out]
      }
    }
  }
